vi "Map Location.vi"(6 "Side":T1=enum."right", 11 "picture":refnum<vi>) -> (0 "error out":errorcluster, 5 "picture":picture)   [LabVIEW 2013]
uses:
  ROS/Code/SubVIs/BaxterSide.ctl
  Teach Locations.ctl
  Baxter Examples/Arm Globals.vi
  <vilib>/Utility/config.llb/Read Key (Double).vi
  <vilib>/Utility/config.llb/Read Key (String).vi
  Move/Move XYA.vi
  Move/Move Joints.vi
  <vilib>/Utility/config.llb/NI_LVConfig.lvlib
panel:
  out "Cluster":T2
  out "Shift":cluster{dbl, dbl, dbl}
  in  "Location Name":string="Mat"
  # "Position gripper over center before starting"
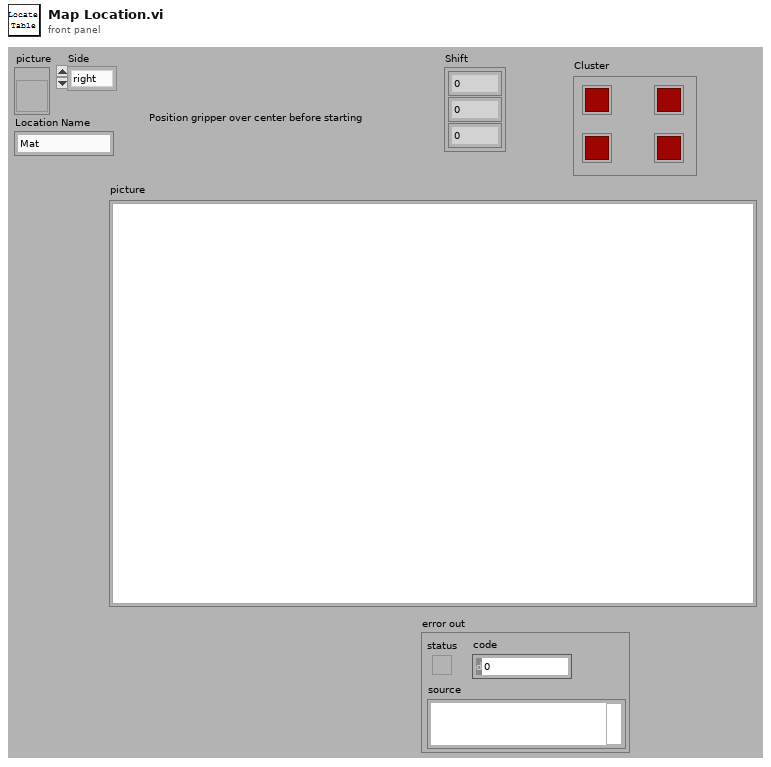
[diagram p1: front panel]
types:
  T1 = typedef "BaxterSide.ctl" = enum16{"left", "right"}
  T2 = cluster{"1":bool, "1 2":bool, "1 3":bool, "1 4":bool}
  T3 = typedef "Teach Locations.ctl" = enum16{"Far_Right", "Near_Right", "Far_Left", "Near_Left", "Bottom", "Top", "Right", "Left"}
  T4 = cluster{"Label":string, "Joints":dbl[], "Far Left":cluster{"Absolute":dbl[], "Robot":dbl[]}, "Far Right":cluster{"Absolute":dbl[], "Robot":dbl[]}, "Near Left":cluster{"Absolute":dbl[], "Robot":dbl[]}, "Near Right":cluster{"Absolute":dbl[], "Robot":dbl[]}}[]
  T5 = typedef "NI_LVConfig.lvlib/Config Data RefNum.ctl" = refnum<k1>
  T6 = cluster{"Label":string, "Joints":dbl[], "Upper Left":cluster{"Absolute":dbl[], "Robot":dbl[]}, "Upper Right":cluster{"Absolute":dbl[], "Robot":dbl[]}, "Lower Left":cluster{"Absolute":dbl[], "Robot":dbl[]}, "Lower Right":cluster{"Absolute":dbl[], "Robot":dbl[]}}
  T7 = cluster{"Label":string, "Joints":dbl[], "Upper Left":cluster{"Absolute":dbl[], "Robot":dbl[]}, "Upper Right":cluster{"Absolute":dbl[], "Robot":dbl[]}, "Lower Left":cluster{"Absolute":dbl[], "Robot":dbl[]}, "Lower Right":cluster{"Absolute":dbl[], "Robot":dbl[]}}[]
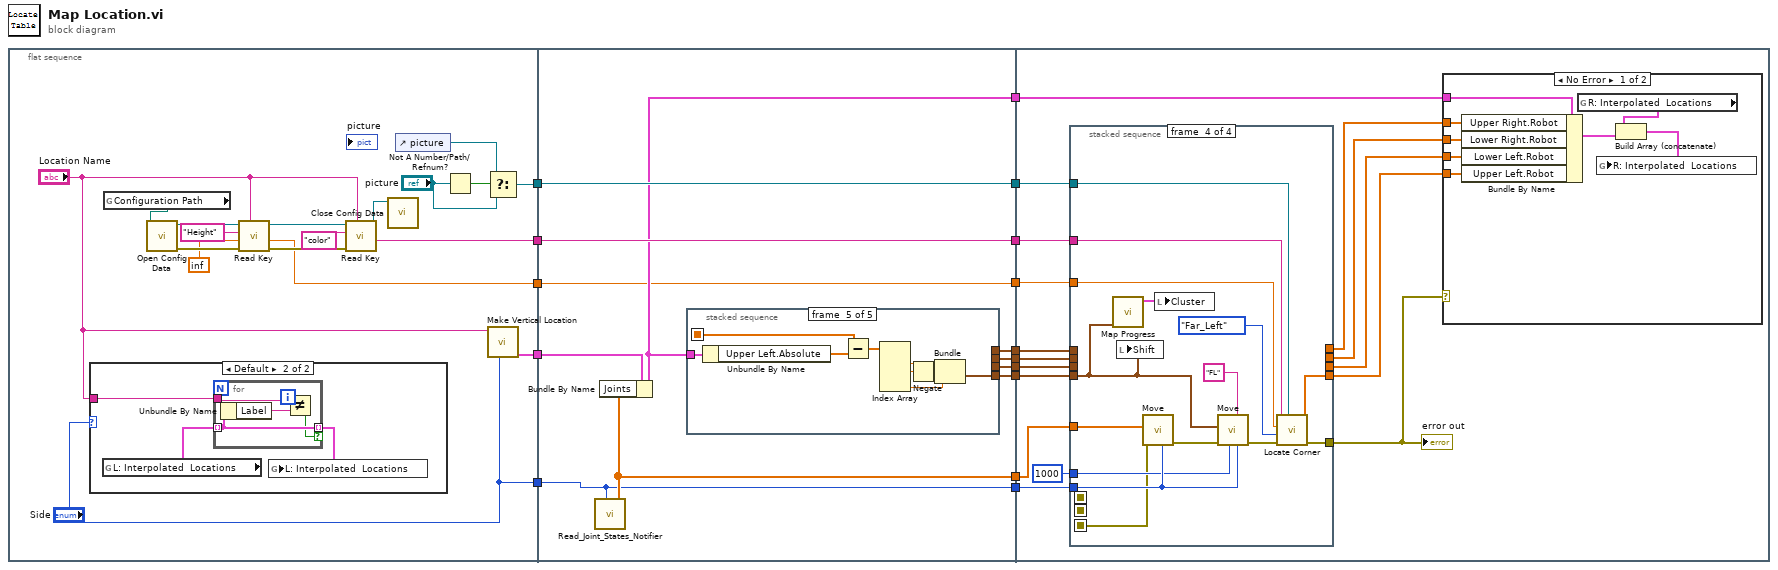
[diagram p0: block diagram]
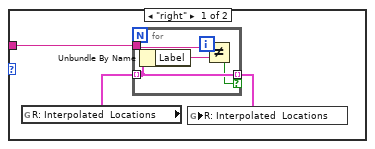
[diagram p2: hidden frame]
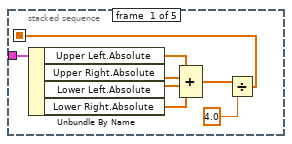
[diagram p3: hidden frame]
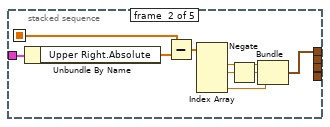
[diagram p4: hidden frame]
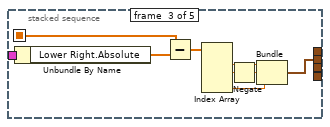
[diagram p5: hidden frame]
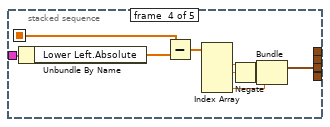
[diagram p6: hidden frame]
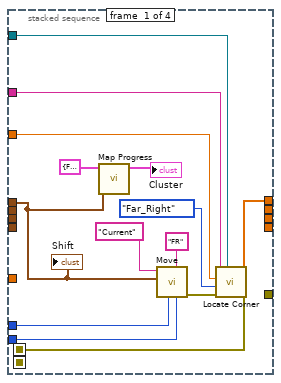
[diagram p7: hidden frame]
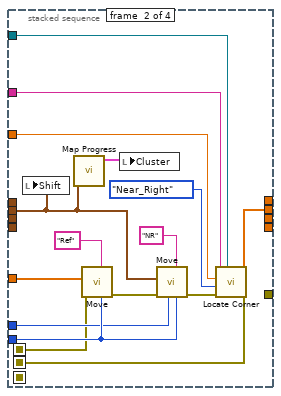
[diagram p8: hidden frame]
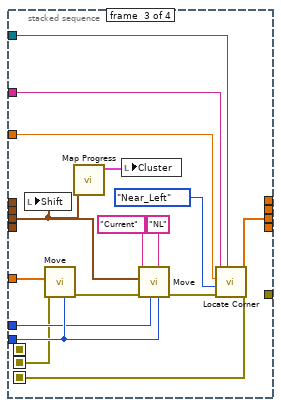
[diagram p9: hidden frame]
diagram:
  n1 = flat-sequence {
    tunnel: [w30] -> w13
    tunnel: [w27] -> w11
    tunnel: [w25] -> w10
    tunnel: ["Side"] -> w3
    tunnel: [w16] -> w2
    tunnel: [w49] -> w15
    tunnel: [w58] -> w14
    tunnel: w13 -> [w58]
    tunnel: [w57] -> w12
    tunnel: w11 -> [w57]
    tunnel: w10 -> [w52]
    tunnel: [w56] -> w9
    tunnel: [w55] -> w8
    tunnel: [w54] -> w7
    tunnel: [w53] -> w6
    tunnel: [w51] -> w5
    tunnel: [w50] -> w4
    tunnel: w3 -> [w49]
    tunnel: w2 -> [w48]
    tunnel: [w48] -> w1
    tunnel: w15 -> [w112]
    tunnel: w14 -> [w114]
    tunnel: w12 -> [w117]
    tunnel: w9 -> [w116]
    tunnel: w8 -> [w110]
    tunnel: w7 -> [w106]
    tunnel: w6 -> [w118]
    tunnel: w5 -> [w109]
    tunnel: w4 -> [w113]
    tunnel: w1 -> [w103]
    frame #0 {
      # "Determine Index Entry in Global \"Locations\" Array"
      n2 = case shown="Default" "Side" {
        tunnel: "Location Name" -> [w34 w41]
        frame "right" {
          n3 = global read "Arm Globals.vi" "R: Interpolated  Locations"() -> (w36:T4)
          n4 = for {
            tunnel: w36 -> [w38] mode=indexing
            tunnel: w34 -> [w39]
            tunnel: [w38] -> w35 mode=indexing if=w37
            n5 = Unbundle By Name(w38) -> ("Label"=w40:string)
            n6 = Not Equal?(x=w39, y=w40) -> (x != y?=w37:bool)
          }
          n7 = global write "Arm Globals.vi" "R: Interpolated  Locations"(w35) -> ()
        }
        frame Default {
          n8 = global read "Arm Globals.vi" "L: Interpolated  Locations"() -> (w43:T4)
          n9 = for {
            tunnel: w43 -> [w45] mode=indexing
            tunnel: w41 -> [w46]
            tunnel: [w45] -> w42 mode=indexing if=w44
            n10 = Unbundle By Name(w45) -> ("Label"=w47:string)
            n11 = Not Equal?(x=w46, y=w47) -> (x != y?=w44:bool)
          }
          n12 = global write "Arm Globals.vi" "L: Interpolated  Locations"(w42) -> ()
        }
      }
      n13 = global read "Arm Globals.vi" "Configuration Path"() -> (w29:path)
      n14 = call <vilib>:"Open Config Data.vi"("configuration file path"=w29) -> ("error out"=w19:errorcluster, "refnum"=w23:T5)  [unwired: 8 in, 1 out]
      n15 = call-poly <vilib>:"Read Key.vi"("section"="Location Name", "error in (no error)"=w19, "default value"=inf, "key"="Height", "refnum"=w23) -> ("error out"=w18:errorcluster, "value"=w16:dbl, "refnum out"=w22:T5)  [unwired: 3 in, 1 out]
      n16 = call-poly <vilib>:"Read Key.vi"("section"="Location Name", "error in (no error)"=w18, "key"="color", "refnum"=w22) -> ("value"=w27:string, "refnum out"=w26:T5)  [unwired: 4 in, 2 out]
      n17 = call <vilib>:"Close Config Data.vi"("refnum"=w26) -> ()  [unwired: 9 in, 2 out]
      n18 = control-ref of="picture"() -> (w31:refnum<vi>)
      n19 = Not A Number/Path/Refnum?(number/path/refnum="picture") -> (NaN/Path/Refnum?=w33:bool)
      n20 = Select(t=w31, s=w33, f="picture") -> (s? t:f=w30:refnum<vi>)
      n21 = call "Make Vertical Location.vi"("Side"="Side", "Location"="Location Name") -> ("Vertical Location"=w25:T6)  [unwired: 9 in]
    }
    frame #1 {
      # "Load Search Pose as Joint Angles\nWill be used to improve repeartability"
      n22 = call "Read_Joint_States_Notifier.vi"("Side"=w49) -> ("Positions"=w50:dbl[])  [unwired: 6 in, 1 out]
      n23 = Bundle By Name(cluster=w52, "Joints"=w50) -> (w53:T6)
      n24 = stacked-sequence {
        seq-local: [w59 _ _ _ _] -> [_ w73 w82 w91 w100]
        tunnel: w53 -> [w66 w75 w84 w93 w102]
        tunnel: [_ _ w77 _ _] -> w56
        tunnel: [_ _ _ w86 _] -> w55
        tunnel: [_ _ _ _ w95] -> w54
        tunnel: [_ w68 _ _ _] -> w51
        frame #0 {
          n25 = Unbundle By Name(w66) -> ("Upper Left.Absolute"=w65:dbl[], "Upper Right.Absolute"=w64:dbl[], "Lower Left.Absolute"=w63:dbl[], "Lower Right.Absolute"=w62:dbl[])
          n26 = Compound Arithmetic op=ADD(w65, w64, w63, w62) -> (w61:dbl[])
          n27 = Divide(x=w61, y=4.0) -> (x/y=w59:dbl[])
        }
        frame #1 {
          n28 = Unbundle By Name(w75) -> ("Upper Right.Absolute"=w74:dbl[])
          n29 = Subtract(x=w73, y=w74) -> (x-y=w72:dbl[])
          n30 = Index Array(array=w72) -> (element #1=w70:dbl, element #2=w71:dbl, element #4=w69:dbl)  [unwired: 4 in, 1 out]
          n31 = Negate(x=w71) -> (-x=w67:dbl)
          n32 = Bundle(w70, w67, w69) -> (w68:cluster{dbl, dbl, dbl})  [unwired: 1 in]
        }
        frame #2 {
          n33 = Unbundle By Name(w84) -> ("Lower Right.Absolute"=w83:dbl[])
          n34 = Subtract(x=w82, y=w83) -> (x-y=w81:dbl[])
          n35 = Index Array(array=w81) -> (element #1=w79:dbl, element #2=w80:dbl, element #4=w78:dbl)  [unwired: 4 in, 1 out]
          n36 = Negate(x=w80) -> (-x=w76:dbl)
          n37 = Bundle(w79, w76, w78) -> (w77:cluster{dbl, dbl, dbl})  [unwired: 1 in]
        }
        frame #3 {
          n38 = Unbundle By Name(w93) -> ("Lower Left.Absolute"=w92:dbl[])
          n39 = Subtract(x=w91, y=w92) -> (x-y=w90:dbl[])
          n40 = Index Array(array=w90) -> (element #1=w88:dbl, element #2=w89:dbl, element #4=w87:dbl)  [unwired: 4 in, 1 out]
          n41 = Negate(x=w89) -> (-x=w85:dbl)
          n42 = Bundle(w88, w85, w87) -> (w86:cluster{dbl, dbl, dbl})  [unwired: 1 in]
        }
        frame #4 {
          n43 = Unbundle By Name(w102) -> ("Upper Left.Absolute"=w101:dbl[])
          n44 = Subtract(x=w100, y=w101) -> (x-y=w99:dbl[])
          n45 = Index Array(array=w99) -> (element #1=w97:dbl, element #2=w98:dbl, element #4=w96:dbl)  [unwired: 4 in, 1 out]
          n46 = Negate(x=w98) -> (-x=w94:dbl)
          n47 = Bundle(w97, w94, w96) -> (w95:cluster{dbl, dbl, dbl})  [unwired: 1 in]
        }
      }
    }
    frame #2 {
      # "Move Arm to allign with the position of the indicator"
      n48 = stacked-sequence {
        seq-local: [w124 _ _ _] -> [_ w139 _ _]
        seq-local: [_ w138 _ _] -> [_ _ w156 _]
        seq-local: [_ _ w155 _] -> [_ _ _ w169]
        tunnel: w117 -> [w130 w144 w162 w176]
        tunnel: w116 -> [_ w134 _ _]
        tunnel: [_ w143 _ _] -> w115
        tunnel: w114 -> [w129 w142 w161 w175]
        tunnel: w113 -> [_ w137 w153 w168]
        tunnel: w112 -> [w128 w141 w160 w174]
        tunnel: [_ _ w159 _] -> w111
        tunnel: w110 -> [_ _ w151 _]
        tunnel: w109 -> [w122 _ _ _]
        tunnel: [w126 _ _ _] -> w108
        tunnel: [_ _ _ w172] -> w107
        tunnel: w106 -> [_ _ _ w167]
        tunnel: [_ _ _ w171] -> w105
        tunnel: 1000 ("wait time") -> [w125 w140 w157 w170]
        tunnel: w103 -> [w119 w133 w149 w165]
        frame #0 {
          n49 = call "Map Progress.vi"("Shift"=w122, "Cluster"=T2 {"1"=FALSE, "1 2"=FALSE, "1 3"=FALSE, "1 4"=FALSE}) -> ("Cluster 2"=→"Cluster":T2)  [unwired: 9 in]
          n50 = call-poly "Move.vi"("Side"=w128, "Label"="FR", "Wait Time"=w125, "XYA"=w122, "Location"="Current") -> ("error out"=w131:errorcluster)  [unwired: 6 in]
          n51 = call "Locate Corner.vi"("picture"=w129, "error in"=w131, "Corner Type"=Teach_Locations."Far_Right" ("Feature"), "Height"=w119, "color"=w130) -> ("error out"=w124:errorcluster, "Robot Point"=w126:dbl[])  [unwired: 4 in, 1 out]
          "Shift" <- w122
        }
        frame #1 {
          n52 = local write "Shift"(w134) -> ()
          n53 = call "Map Progress.vi"("Shift"=w134) -> ("Cluster 2"=w135:T2)  [unwired: 10 in]
          n54 = call-poly "Move.vi"("Side"=w141, "Label"="Ref", "error in"=w139, "Goal"=w137) -> ("error out"=w148:errorcluster)  [unwired: 7 in]
          n55 = local write "Cluster"(w135) -> ()
          n56 = call-poly "Move.vi"("Side"=w141, "Label"="NR", "Wait Time"=w140, "error in"=w148, "XYA"=w134) -> ("error out"=w146:errorcluster)  [unwired: 6 in]
          n57 = call "Locate Corner.vi"("picture"=w142, "error in"=w146, "Corner Type"=Teach_Locations."Near_Right", "Height"=w133, "color"=w144) -> ("error out"=w138:errorcluster, "Robot Point"=w143:dbl[])  [unwired: 4 in, 1 out]
        }
        frame #2 {
          n58 = local write "Shift"(w151) -> ()
          n59 = call-poly "Move.vi"("Side"=w160, "error in"=w156, "Goal"=w153) -> ("error out"=w164:errorcluster)  [unwired: 8 in]
          n60 = call "Map Progress.vi"("Shift"=w151) -> ("Cluster 2"=w150:T2)  [unwired: 10 in]
          n61 = local write "Cluster"(w150) -> ()
          n62 = call-poly "Move.vi"("Side"=w160, "Label"="NL", "Wait Time"=w157, "error in"=w164, "XYA"=w151, "Location"="Current") -> ("error out"=w163:errorcluster)  [unwired: 5 in]
          n63 = call "Locate Corner.vi"("picture"=w161, "error in"=w163, "Corner Type"=Teach_Locations."Near_Left", "Height"=w149, "color"=w162) -> ("error out"=w155:errorcluster, "Robot Point"=w159:dbl[])  [unwired: 4 in, 1 out]
        }
        frame #3 {
          n64 = call "Map Progress.vi"("Shift"=w167) -> ("Cluster 2"=w166:T2)  [unwired: 10 in]
          n65 = local write "Shift"(w167) -> ()
          n66 = call-poly "Move.vi"("Side"=w174, "error in"=w169, "Goal"=w168) -> ("error out"=w179:errorcluster)  [unwired: 8 in]
          n67 = local write "Cluster"(w166) -> ()
          n68 = call-poly "Move.vi"("Side"=w174, "Label"="FL", "Wait Time"=w170, "error in"=w179, "XYA"=w167) -> ("error out"=w177:errorcluster)  [unwired: 6 in]
          n69 = call "Locate Corner.vi"("picture"=w175, "error in"=w177, "Corner Type"=Teach_Locations."Far_Left", "Height"=w165, "color"=w176) -> ("error out"=w171:errorcluster, "Robot Point"=w172:dbl[])  [unwired: 4 in, 1 out]
        }
      }
      "error out" <- w105
      n70 = case shown="No Error" w105 {
        tunnel: w118 -> [w187 _]
        tunnel: w108 -> [w186 _]
        tunnel: w115 -> [w185 _]
        tunnel: w111 -> [w184 _]
        tunnel: w107 -> [w183 _]
        frame No Error {
          n71 = Bundle By Name(cluster=w187, "Upper Right.Robot"=w186, "Lower Right.Robot"=w185, "Lower Left.Robot"=w184, "Upper Left.Robot"=w183) -> (w180:T6)
          n72 = global read "Arm Globals.vi" "R: Interpolated  Locations"() -> (w182:T4)
          n73 = Build Array (concatenate)(w182, w180) -> (w181:T7)
          n74 = global write "Arm Globals.vi" "R: Interpolated  Locations"(w181) -> ()
        }
        frame Error {
        }
      }
    }
  }
